vi "BonOMM-SAOMM.vi"() -> ()   [LabVIEW 2019] (continued)
          n252 = property on="Saturé" class="Bool (strict)"("Visible"=w229, "Blinking"=w229) -> ()  [unwired: 2 in, 2 out]
          n253 = call-poly <vilib>:"Read Key.vi"("section"=w271, "error in (no error)"=w284, "key"="DefaultROIOffset", "refnum"=w285) -> ("error out"=w276:errorcluster, "value"=w277:u32, "refnum out"=w275:T23)  [unwired: 4 in, 1 out]
          n254 = To Unsigned Word Integer(number=w333) -> (unsigned 16bit integer=w334:u16)
          n255 = To Unsigned Word Integer(number=w332) -> (unsigned 16bit integer=w331:u16)
          n256 = local write "ROIHeight"(w334) -> ()
          n257 = local write "ROIWidth"(w331) -> ()
          n258 = property on="TableXYPos" class="GraphXY (strict)"(error in=w535, "Active Cursor"=u32 1) -> (error out=w533:errorcluster)  [unwired: 1 in, 1 out]
          n259 = call-poly <vilib>:"Read Key.vi"("section"=w271, "error in (no error)"=w276, "key"="DefaultBinning", "refnum"=w275) -> ("error out"=w265:errorcluster, "value"=w278:u32, "refnum out"=w266:T23)  [unwired: 4 in, 1 out]
          n260 = call-poly <vilib>:"Read Key.vi"("section"=w260, "error in (no error)"=w265, "key"="GuideRateRA", "refnum"=w266) -> ("error out"=w351:errorcluster, "value"=w342:dbl, "refnum out"=w352:T23)  [unwired: 4 in, 1 out]
          n261 = local write "RateRA"(w342) -> ()
          n262 = call-poly <vilib>:"Read Key.vi"("section"=w260, "error in (no error)"=w351, "key"="GuideRateDEC", "refnum"=w352) -> ("error out"=w258:errorcluster, "value"=w341:dbl, "refnum out"=w259:T23)  [unwired: 4 in, 1 out]
          n263 = local write "RateDEC"(w341) -> ()
          n264 = call-poly <vilib>:"Read Key.vi"("section"=w260, "error in (no error)"=w258, "key"="HexXRate", "refnum"=w259) -> ("error out"=w264:errorcluster, "value"=w255:dbl, "refnum out"=w263:T23)  [unwired: 4 in, 1 out]
          n265 = local write "HexXRate"(w255) -> ()
          n266 = call-poly <vilib>:"Read Key.vi"("section"=w260, "error in (no error)"=w264, "key"="HexYRate", "refnum"=w263) -> ("error out"=w256:errorcluster, "value"=w254:dbl, "refnum out"=w257:T23)  [unwired: 4 in, 1 out]
          n267 = local write "HexYRate"(w254) -> ()
          n268 = call-poly <vilib>:"Read Key.vi"("section"=w260, "error in (no error)"=w256, "key"="BacklashRA", "refnum"=w257) -> ("error out"=w350:errorcluster, "value"=w340:dbl, "refnum out"=w353:T23)  [unwired: 4 in, 1 out]
          n269 = local write "BacklashRA"(w340) -> ()
          n270 = call-poly <vilib>:"Read Key.vi"("section"=w260, "error in (no error)"=w350, "key"="BacklashDEC", "refnum"=w353) -> ("error out"=w357:errorcluster, "value"=w339:dbl, "refnum out"=w356:T23)  [unwired: 4 in, 1 out]
          n271 = local write "BacklashDEC"(w339) -> ()
          n272 = call-poly <vilib>:"Read Key.vi"("section"=w260, "error in (no error)"=w357, "key"="GuiderAgg", "refnum"=w356) -> ("error out"=w355:errorcluster, "value"=w343:dbl, "refnum out"=w354:T23)  [unwired: 4 in, 1 out]
          n273 = local write "Corr%"(w343) -> ()
          n274 = call-poly <vilib>:"Read Key.vi"("section"=w260, "error in (no error)"=w355, "key"="GuiderTreshold", "refnum"=w354) -> ("error out"=w346:errorcluster, "value"=w344:dbl, "refnum out"=w347:T23)  [unwired: 4 in, 1 out]
          n275 = local write "CorrTreshold"(w344) -> ()
          n276 = call-poly <vilib>:"Read Key.vi"("section"=w260, "error in (no error)"=w346, "key"="SNRTreshold", "refnum"=w347) -> ("error out"=w267:errorcluster, "value"=→"SNRtreshold":dbl, "refnum out"=w268:T23)  [unwired: 4 in, 1 out]
          n277 = call-poly <vilib>:"Read Key.vi"("section"=w269, "error in (no error)"=w267, "key"="UAxisOffset", "refnum"=w268) -> ("error out"=w292:errorcluster, "value"=w287:dbl, "refnum out"=w293:T23)  [unwired: 4 in, 1 out]
          n278 = local write "DefaultUAxisOffset"(w287) -> ()
          n279 = call-poly <vilib>:"Read Key.vi"("section"=w269, "error in (no error)"=w292, "key"="VAxisOffset", "refnum"=w293) -> ("error out"=w290:errorcluster, "value"=w286:dbl, "refnum out"=w291:T23)  [unwired: 4 in, 1 out]
          n280 = local write "DefaultVAxisOffset"(w286) -> ()
          n281 = call-poly <vilib>:"Read Key.vi"("section"=w269, "error in (no error)"=w290, "key"="Sampling", "refnum"=w291) -> ("error out"=w327:errorcluster, "value"=→"Sampling rate":i32, "refnum out"=w328:T23)  [unwired: 4 in, 1 out]
          n282 = call-poly <vilib>:"Read Key.vi"("section"=w269, "error in (no error)"=w327, "key"="DataLenght", "refnum"=w328) -> ("error out"=w249:errorcluster, "value"=w345:i32, "refnum out"=w248:T23)  [unwired: 4 in, 1 out]
          n283 = local write "ConsideredLenght"(w345) -> ()
          n284 = local write "Flat"(w484) -> ()
          n285 = call-poly <vilib>:"Read Key.vi"("section"=w221, "error in (no error)"=w249, "key"="PRAMMS-SG", "refnum"=w248) -> ("error out"=w227:errorcluster, "value"=w246:u32, "refnum out"=w228:T23)  [unwired: 4 in, 1 out]
          n286 = property on="TableXYPos" class="GraphXY (strict)"(error in=w533, "Cursor.Cursor X"=w529, "Cursor.Cursor Y"=w529) -> ()  [unwired: 1 in, 2 out]
          n287 = local write "Néon"(w484) -> ()
          n288 = local write "Signature"(w246) -> ()
          n289 = To Unsigned Word Integer(number=w278) -> (unsigned 16bit integer=w279:u16)
          n290 = To Unsigned Word Integer(number=w277) -> (unsigned 16bit integer=w281:u16)
          n291 = To Unsigned Word Integer(number=w277) -> (unsigned 16bit integer=w280:u16)
          n292 = local write "Arc"(w484) -> ()
          n293 = local write "Binning"(w279) -> ()
          n294 = local write "ROIYOffset"(w281) -> ()
          n295 = local write "ROIXOffset"(w280) -> ()
          n296 = local write "NeonOn"(w484) -> ()
          n297 = local write "ArcOn"(w484) -> ()
          n298 = global read "Globals.vi" "BonOMM VI Refnum"() -> (w294:refnum<vi>)
          n299 = call-poly <vilib>:"Read Key.vi"("section"=w221, "error in (no error)"=w227, "key"="tempspd", "refnum"=w228) -> ("error out"=w224:errorcluster, "value"=w218:u32, "refnum out"=w225:T23)  [unwired: 4 in, 1 out]
          n300 = local write "FlatOn"(w484) -> ()
          n301 = Initialize Array(0.0, 0) -> (w252:dbl[])
          n302 = Initialize Array(sgl 0.0, w527, w527) -> (w526:sgl[][])
          n303 = Bundle(w424, w424, w424) -> (w423:cluster{string, string, string})  [unwired: 1 in]
          n304 = local write "ImgData"(w526) -> ()
          n305 = local write "MC_connect"(FALSE) -> ()
          n306 = call-poly <vilib>:"Read Key.vi"("section"=w221, "error in (no error)"=w224, "key"="tempvrn", "refnum"=w225) -> ("error out"=w222:errorcluster, "value"=w219:string, "refnum out"=w223:T23)  [unwired: 4 in, 1 out]
          n307 = call-poly <vilib>:"Read Key.vi"("section"=w313, "error in (no error)"=w222, "key"="xgain", "refnum"=w223) -> ("error out"=w320:errorcluster, "value"=→"Gain X":dbl, "refnum out"=w319:T23)  [unwired: 4 in, 1 out]
          n308 = call-poly <vilib>:"Read Key.vi"("section"=w313, "error in (no error)"=w320, "key"="ygain", "refnum"=w319) -> ("error out"=w315:errorcluster, "value"=→"Gain Y":dbl, "refnum out"=w316:T23)  [unwired: 4 in, 1 out]
          n309 = call-poly <vilib>:"Read Key.vi"("section"=w313, "error in (no error)"=w315, "key"="zgain", "refnum"=w316) -> ("error out"=w325:errorcluster, "value"=→"Gain Z":dbl, "refnum out"=w324:T23)  [unwired: 4 in, 1 out]
          n310 = call-poly <vilib>:"Read Key.vi"("section"=w313, "error in (no error)"=w325, "key"="ugain", "refnum"=w324) -> ("error out"=w323:errorcluster, "value"=→"Gain U":dbl, "refnum out"=w322:T23)  [unwired: 4 in, 1 out]
          n311 = call-poly <vilib>:"Read Key.vi"("section"=w313, "error in (no error)"=w323, "key"="vgain", "refnum"=w322) -> ("error out"=w273:errorcluster, "value"=→"Gain V":dbl, "refnum out"=w274:T23)  [unwired: 4 in, 1 out]
          n312 = call-poly <vilib>:"Read Key.vi"("section"="options", "error in (no error)"=w273, "default value"=FALSE, "key"="autoconnect", "refnum"=w274) -> ("error out"=w389:errorcluster, "value"=w385:bool, "refnum out"=w390:T23)  [unwired: 3 in, 1 out]
          n313 = local write "AutoConnect?"(w385) -> ()
          n314 = call-poly <vilib>:"Read Key.vi"("section"=w393, "error in (no error)"=w389, "key"="secperpulse", "refnum"=w390) -> ("error out"=w403:errorcluster, "value"=w242:dbl, "refnum out"=w405:T23)  [unwired: 4 in, 1 out]
          "arcsec/pulse" <- w242
          n315 = call-poly <vilib>:"Read Key.vi"("section"=w393, "error in (no error)"=w403, "key"="naxis1", "refnum"=w405) -> ("error out"=w402:errorcluster, "value"=w243:dbl, "refnum out"=w404:T23)  [unwired: 4 in, 1 out]
          n316 = local write "NaxisMax"(w243) -> ()
          n317 = Multiply(x=w243, y=w242) -> (x*y=w241:dbl)
          n318 = call-poly <vilib>:"Read Key.vi"("section"=w393, "error in (no error)"=w402, "key"="represent", "refnum"=w404) -> ("error out"=w434:errorcluster, "value"=w431:dbl, "refnum out"=w435:T23)  [unwired: 4 in, 1 out]
          "Représentation" <- w431
          n319 = expression code="x/60"(w241) -> (→"RangeTable":dbl)
          n320 = call-poly <vilib>:"Read Key.vi"("section"=w393, "error in (no error)"=w434, "key"="cenx", "refnum"=w435) -> ("error out"=w516:errorcluster, "value"=w515:i32, "refnum out"=w517:T23)  [unwired: 4 in, 1 out]
          n321 = local write "CentreTel X"(w515) -> ()
          n322 = call-poly <vilib>:"Read Key.vi"("section"=w393, "error in (no error)"=w516, "key"="ceny", "refnum"=w517) -> ("error out"=w508:errorcluster, "value"=w514:i32, "refnum out"=w509:T23)  [unwired: 4 in, 1 out]
          n323 = local write "CentreTel Y"(w514) -> ()
          n324 = call-poly <vilib>:"Read Key.vi"("section"=w393, "error in (no error)"=w508, "key"="refx", "refnum"=w509) -> ("error out"=w513:errorcluster, "value"=w507:i32, "refnum out"=w512:T23)  [unwired: 4 in, 1 out]
          n325 = local write "Reference X"(w507) -> ()
          n326 = call-poly <vilib>:"Read Key.vi"("section"=w393, "error in (no error)"=w513, "key"="refy", "refnum"=w512) -> ("error out"=w444:errorcluster, "value"=w506:i32, "refnum out"=w445:T23)  [unwired: 4 in, 1 out]
          n327 = local write "Reference Y"(w506) -> ()
          n328 = Less Or Equal?(x=w431, y=70.0) -> (x <= y?=w429:bool)
          n329 = call-poly <vilib>:"Read Key.vi"("section"=w393, "error in (no error)"=w444, "key"="rangex", "refnum"=w445) -> ("error out"=w446:errorcluster, "value"=w449:i32, "refnum out"=w447:T23)  [unwired: 4 in, 1 out]
          n330 = local write "Rangement X"(w449) -> ()
          n331 = Select(t=T17."Enabled" ("Disabled"), s=w429, f=T17."Disabled" ("Disabled")) -> (s? t:f=w426:T17)
          n332 = call-poly <vilib>:"Read Key.vi"("section"=w393, "error in (no error)"=w446, "key"="rangey", "refnum"=w447) -> ("error out"=w440:errorcluster, "value"=w450:i32, "refnum out"=w441:T23)  [unwired: 4 in, 1 out]
          n333 = local write "Rangement Y"(w450) -> ()
          n334 = property on="GetDSS" class="Bool (strict)"("DisabledEnum"=w426) -> ()  [unwired: 2 in, 2 out]
          n335 = call-poly <vilib>:"Read Key.vi"("section"=w393, "error in (no error)"=w440, "key"="rangez", "refnum"=w441) -> ("error out"=w438:errorcluster, "value"=w437:i32, "refnum out"=w439:T23)  [unwired: 4 in, 1 out]
          n336 = local write "Rangement Z"(w437) -> ()
          n337 = call-poly <vilib>:"Read Key.vi"("section"=w393, "error in (no error)"=w438, "key"="vrapid", "refnum"=w439) -> ("error out"=w476:errorcluster, "value"=→"vitesse rapide":dbl, "refnum out"=w475:T23)  [unwired: 4 in, 1 out]
          n338 = call-poly <vilib>:"Read Key.vi"("section"=w393, "error in (no error)"=w476, "key"="vlente", "refnum"=w475) -> ("error out"=w482:errorcluster, "value"=→"vitesse lente":dbl, "refnum out"=w481:T23)  [unwired: 4 in, 1 out]
          n339 = call-poly <vilib>:"Read Key.vi"("section"=w393, "error in (no error)"=w482, "key"="accel", "refnum"=w481) -> ("error out"=w477:errorcluster, "value"=→"accelleration":dbl, "refnum out"=w478:T23)  [unwired: 4 in, 1 out]
          n340 = call-poly <vilib>:"Read Key.vi"("section"=w393, "error in (no error)"=w477, "key"="vfocus", "refnum"=w478) -> ("error out"=w396:errorcluster, "value"=→"vitesse focus":dbl, "refnum out"=w397:T23)  [unwired: 4 in, 1 out]
          n341 = call-poly <vilib>:"Read Key.vi"("section"=w393, "error in (no error)"=w396, "key"="vjog", "refnum"=w397) -> ("error out"=w394:errorcluster, "value"=→"vitesse jog":dbl, "refnum out"=w395:T23)  [unwired: 4 in, 1 out]
          n342 = call <vilib>:"Close Config Data.vi"("error in (no error)"=w394, "refnum"=w395) -> ("file path"=w454:path)  [unwired: 8 in, 1 out]
          n343 = call "Readwindowpropfile.vi"("configuration file path"=w454) -> ("PanelOrigin"=w296:cluster{"panelx":i16, "panely":i16}, "MinimumSize"=w297:cluster{"Horizontal":i16, "Vertical":i16}, "PanelBounds"=w298:T24, "resizable"=w299:bool, "AllFound"=w295:bool)  [unwired: 6 in]
          n344 = Bundle(w252, w252) -> (w460:cluster{dbl[], dbl[]})  [unwired: 1 in]
          n345 = Initialize Array(w423, 0) -> (→"CmdDone":cluster{string, string, string}[])
          n346 = flat-sequence {
            tunnel: w294 -> [w569]
            tunnel: w299 -> [w570]
            tunnel: w298 -> [w571]
            tunnel: w297 -> [w565]
            tunnel: [w572] -> w306
            tunnel: w296 -> [w572]
            tunnel: [w568] -> w305
            tunnel: [w571] -> w304
            tunnel: [w570] -> w303
            tunnel: [w566] -> w302
            tunnel: [w565] -> w301
            tunnel: w306 -> [w578]
            tunnel: [w578] -> w300
            tunnel: w305 -> [w577]
            tunnel: w304 -> [w576]
            tunnel: w303 -> [_]
            tunnel: w302 -> [w575]
            tunnel: w301 -> [w574]
            tunnel: w300 -> [w584]
            frame #0 {
              n347 = property class="VI"(reference=w569, "Front Panel.Resizeable"=TRUE ("Front Panel Window:Resizable")) -> (reference out=w568:refnum<vi>, error out=w566:errorcluster)  [unwired: 1 in]
            }
            frame #1 {
              n348 = disable-structure shown="Disabled" {
                disable-tunnel: w577 -> [w583 _]
                disable-tunnel: w576 -> [w582 _]
                disable-tunnel: w575 -> [w581 _]
                disable-tunnel: w574 -> [w580 _]
                disable-tunnel: TRUE ("Front Panel Window:Resizable") -> [w579 _]
                frame Disabled {
                  n349 = property class="VI"(reference=w583, error in=w581, "Front Panel.Resizeable"=w579, "Front Panel.PanelBounds"=w582, "Minimum Panel Size"=w580) -> ()  [unwired: 2 out]
                }
                frame Enabled {
                }
              }
            }
            frame #2 {
              n350 = property on="Pane" class="Pann"("Origin"=w584) -> ()  [unwired: 2 in, 2 out]
              n351 = property on="MainTab" class="Onglet (strict)"("Position"=cluster{i32, i32} {0, 0}) -> ()  [unwired: 2 in, 2 out]
            }
            frame #3 {
              "Lecture Configuration" <- TRUE ("Lecture Configuration")
            }
          }
          n352 = case shown="Vrai" w295 {
            frame False {
              # "Ne devrais pas arriver ..."
              n353 = One Button Dialog(message="Impossible de trouver le fichier properties.ini\nUtilisation des valeurs par défauts ...") -> ()  [unwired: 1 in, 1 out]
            }
            frame True {
            }
          }
          n354 = local write "LVDT-RA-Data"(w252) -> ()
          n355 = call "Draw_crosshair.vi"("Image IN"=w526, "White Value"=sgl 255.0) -> ("Image OUT"=w525:sgl[][])  [unwired: 13 in]
          n356 = Initialize Array(w460, 0) -> (w253:cluster{dbl[], dbl[]}[])
          n357 = Initialize Array("", 0) -> (w469:string[])
          n358 = Initialize Array(refnum<k5> refnum ("External TCP ID 2"), 0) -> (w467:refnum<k5>[])
          n359 = local write "subimg"(w525) -> ()
          n360 = local write "Img DEC"(w436) -> ()
          n361 = local write "RA-USNO"(w436) -> ()
          n362 = local write "DEC-USNO"(w436) -> ()
          n363 = local write "Img RA"(w436) -> ()
          n364 = local write "Graph-Flux"(w253) -> ()
          n365 = local write "Graph-Centroids"(w253) -> ()
          n366 = local write "Graph-SNR"(w253) -> ()
          n367 = local write "ImageUsage"(w384) -> ()
          n368 = disable-structure shown="Activé" {
            disable-tunnel: w219 -> [w563 _]
            disable-tunnel: w218 -> [w562 _]
            frame Disabled {
              n369 = Type Cast(type=refnum<visa-resource-name> "-1" ("Table VRN"), x=w563) -> (*(type *) &x=w557:refnum<visa-resource-name>)
              n370 = local write "HexTemp Baud rate"(w562) -> ()
              n371 = local write "HexTemp VRN"(w557) -> ()
              n372 = call-poly "VISA Configure Serial Port"("VISA resource name"=w557, "timeout (10sec)"=u32 1000, "Enable Termination\nChar (T)"=FALSE ("Enable Termination\nChar (T)"), "baud rate (9600)"=w562) -> ("error out"=w558:errorcluster)  [unwired: 10 in, 1 out]
              n373 = local write "HexapodeTempError"(w558) -> ()
            }
            frame Enabled {
            }
          }
          n374 = local write "Clients ID"(w467) -> ()
          n375 = local write "Clients"(w469) -> ()
          n376 = local write "Hex-XGraph"(w253) -> ()
          n377 = local write "Guiderreur"(w253) -> ()
          n378 = local write "Hex-YGraph"(w253) -> ()
          n379 = local write "Cumulatif"(w253) -> ()
          n380 = local write "CumulativeError"(w253) -> ()
          n381 = local write "CentroidsData"(w253) -> ()
          n382 = local write "HexXData"(w253) -> ()
          n383 = local write "HexYData"(w253) -> ()
          n384 = local write "SNRData"(w253) -> ()
          n385 = local write "FluxData"(w253) -> ()
          "RAtmp" <- w436
          "Dectmp" <- w436
          "Menu Error" <- w472
          "VI Reference Error" <- w472
          "Starry Night Error" <- w472
          "Excom Error" <- w472
          "Guider Error" <- w472
          "ActiveX Error" <- w472
          "Critical Error" <- w472
          "Config Error" <- w472
          "Serial Error" <- w472
          "TCP/IP Error" <- w472
          "wget error" <- w472
          "TCS Error" <- w472
          "File I/O Error" <- w472
          "FIFO actif" <- w244
          "TCS actif" <- w244
          "TCS C actif" <- w244
          "Table actif" <- w244
          "Integrating" <- w244
          "MovingXY" <- w244
          "MovingZ" <- w244
          "CorrectZ" <- w244
          "CorrectXY" <- w244
          "Focusing" <- w244
          "CurvCorrect" <- w244
          "SubIMG4DSS?" <- w244
          "AS_I_Pillier" <- FALSE ("AS_Pillier")
          "GE_TCS" <- FALSE ("GE_TCS")
        }
      }
      n386 = property on="Déc étoile guide" class="NumNb (strict)"("Visible"=w201) -> ()  [unwired: 2 in, 2 out]
      n387 = property on="A.D. étoile guide" class="NumNb (strict)"("Visible"=w201) -> ()  [unwired: 2 in, 2 out]
      n388 = property on="Graph-Centroids" class="GraphXY (strict)"("Visible"=w201) -> ()  [unwired: 2 in, 2 out]
      n389 = property on="Flux Max" class="NumNb (strict)"("Visible"=w201) -> ()  [unwired: 2 in, 2 out]
      n390 = property on="Guiderreur" class="GraphXY (strict)"("Visible"=w201) -> ()  [unwired: 2 in, 2 out]
      n391 = property on="Flux inst." class="NumNb (strict)"("Visible"=w201) -> ()  [unwired: 2 in, 2 out]
      n392 = property on="StopCam" class="Bool (strict)"("Visible"=w201) -> ()  [unwired: 2 in, 2 out]
      n393 = property on="GoCam" class="Bool (strict)"("Visible"=w201) -> ()  [unwired: 2 in, 2 out]
      n394 = property on="Approaching limit" class="Bool (strict)"("Visible"=w203, "Blinking"=w203) -> ()  [unwired: 2 in, 2 out]
      n395 = property on="Target OutofRange" class="Bool (strict)"("Visible"=w203, "Blinking"=w203) -> ()  [unwired: 2 in, 2 out]
      n396 = property on="Lampe Allumée ?" class="Bool (strict)"("Visible"=w203, "Blinking"=w203) -> ()  [unwired: 2 in, 2 out]
      n397 = property on="ModeInv" class="Bool (strict)"("Visible"=w203, "Blinking"=w203) -> ()  [unwired: 2 in, 2 out]
      n398 = property on="StarFaded?" class="Bool (strict)"("Visible"=w203, "Blinking"=w203) -> ()  [unwired: 2 in, 2 out]
      n399 = property on="Alarme PRAMS" class="Bool (strict)"("Visible"=w203, "Blinking"=w203) -> ()  [unwired: 2 in, 2 out]
      n400 = property on="Picture" class="Image"("Visible"=w202) -> ()  [unwired: 2 in, 2 out]
      n401 = property on="filtre_nom" class="Ch"("Visible"=w202) -> ()  [unwired: 2 in, 2 out]
      n402 = property on="q-raf" class="Bool (strict)"("Visible"=w202) -> ()  [unwired: 2 in, 2 out]
      n403 = property on="cancel-raf" class="Bool (strict)"("Visible"=w202) -> ()  [unwired: 2 in, 2 out]
      n404 = property on="change_filtre_liste" class="Bool (strict)"("Visible"=w202) -> ()  [unwired: 2 in, 2 out]
      n405 = property on="ChoixFiltre" class="Clust (strict)"("Visible"=w202) -> ()  [unwired: 2 in, 2 out]
      n406 = property on="F#" class="NumNb (strict)"("Visible"=w202) -> ()  [unwired: 2 in, 2 out]
      n407 = property on="ST-" class="Bool (strict)"("Visible"=w202) -> ()  [unwired: 2 in, 2 out]
      n408 = property on="ST+" class="Bool (strict)"("Visible"=w202) -> ()  [unwired: 2 in, 2 out]
      n409 = property on="SET ZERO" class="Bool"("Visible"=w202) -> ()  [unwired: 2 in, 2 out]
      n410 = property on="ST_RAZ" class="Bool"("Visible"=w202) -> ()  [unwired: 2 in, 2 out]
      n411 = property on="reconnect" class="Bool (strict)"("Visible"=w202) -> ()  [unwired: 2 in, 2 out]
      n412 = property on="ST_SPD" class="Gliss (strict)"("Visible"=w202) -> ()  [unwired: 2 in, 2 out]
      "GE_Hex_X" <- w200
      "GE_Hex_Y" <- w200
      "GE_Hex_Z" <- w200
      "GE_Hex_U" <- w200
      "GE_Hex_V" <- w200
    }
    frame #4 {
      # "Étape 4 de l'initialisation"
      # "Initialisation des éléments du menu"
      n413 = case shown="Vrai" w587 {
        frame False {
        }
        frame True {
          w671 = refnum<visa-resource-name> "-1" ("Table VRN")
          # "Menu \"FA (Fonctions avancées)\""
          # "Désactive les filtres"
          # "Menu \"Roue à filtre\""
          # "Menu \"Tables de guidage\""
          # "Menu \"Caméra de référence\""
          # "Menu \"Secondaire Actif\""
          # "Menu \"Télescope\""
          # "Menu des scripts"
          # "Menu des Instruments"
          # "Menu des communications"
          # "Ajoute les items de menu custom"
          # "Enlève les items de menu non-utilisés"
          n414 = Current VI's Menubar ("Barre de menu")() -> (w715:refnum<k9>)
          n415 = Delete Menu Items(7:string[] ["APP_EDIT", "APP_VIEW", "APP_PROJECT", "APP_TOOLS"], 9:w715) -> (0:w673:errorcluster, 3:w674:refnum<k9>)  [unwired: 2 in]
          n416 = call "MenuFixer.vi"("Menu Name"=string[] ["Communications", "Instruments", "Scripts et Automatismes", "Télescope", "Secondaire Actif", "Caméra de référence", "Tables de guidage", "Roue à filtres", "FA"] ("Array Constant"), "Prefix"="main_") -> ("Item Tags"=w614:string[], "Item Names"=w613:string[])  [unwired: 8 in]
          n417 = call "MenuFixer.vi"("Menu Name"=string[] ["Charger la librairie CPAPIR", "Charger la librairie Pesto", "Charger une librairie d'objets", "APP_SEPARATOR", "Déterminer l'astrométrie du champ", "Calibration du foyer automatique", "APP_SEPARATOR", "Construction d'une LUT"] ("menuelem_cmd"), "Prefix"="scp_") -> ("Item Tags"=w626:string[], "Item Names"=w625:string[])  [unwired: 8 in]
          n418 = Insert Menu Items(4:"APP_OPERATE" ("after item"), 6:w673, 7:w614, 8:w613, 9:w674) -> (0:w664:errorcluster, 3:w665:refnum<k9>)  [unwired: 1 in, 1 out]
          n419 = call "MenuFixer.vi"("Menu Name"=string[] ["Telescope Control System", "Caméra de référence", "Tables de guidage", "Secondaire Actif", "Module de calibration", "MC-BonOMM", "Commandes externes", "Station Météo", "APP_SEPARATOR", "Reconnexion automatique ?"] ("menu_comm"), "Prefix"="com_") -> ("Item Tags"=w612:string[], "Item Names"=w618:string[])  [unwired: 8 in]
          n420 = Insert Menu Items(5:"main_Communications" ("menu tag"), 6:w664, 7:w612, 8:w618, 9:w665) -> (0:w707:errorcluster, 3:w708:refnum<k9>)  [unwired: 1 in, 1 out]
          n421 = call "MenuFixer.vi"("Menu Name"=string[] ["Synchroniser la coupole", "Synchroniser les horloges", "Modifier la vitesse du télescope", "Modifier la vitesse de guidage", "Modifier l'époque d'affichage", "Test signal vers TCS ", "APP_SEPARATOR", "Reconnexion"] ("menuelem_cmd"), "Prefix"="tel_") -> ("Item Tags"=w631:string[], "Item Names"=w630:string[])  [unwired: 8 in]
          n422 = Index Array(array=w612) -> (element #1=w698:string, element #2=w697:string, element #3=w696:string, element #4=w666:string, element #5=w679:string, element #6=w678:string, element #7=w677:string, element #8=w676:string, element #10=w675:string)  [unwired: 10 in, 1 out]
          n423 = local read "TCS VRN"() -> (w704:refnum<visa-resource-name>)
          n424 = Not Equal?(x=w704, y=w671) -> (x != y?=w689:bool)
          n425 = local write "TCS COMM"(w689) -> ()
          n426 = Set Menu Item Info(6:w689, 7:w698, 8:w707, 11:w708) -> (0:w710:errorcluster, 3:w709:refnum<k9>)  [unwired: 3 in]
          n427 = local read "PrAMS VRN"() -> (w703:refnum<visa-resource-name>)
          n428 = Not Equal?(x=w703, y=w671) -> (x != y?=w688:bool)
          n429 = local write "PrAMS COMM"(w688) -> ()
          n430 = Set Menu Item Info(6:w688, 7:w697, 8:w710, 11:w709) -> (0:w712:errorcluster, 3:w711:refnum<k9>)  [unwired: 3 in]
          n431 = local read "Table VRN"() -> (w702:refnum<visa-resource-name>)
          n432 = call "MenuFixer.vi"("Menu Name"=string[] ["Paramètres d'asservissement", "Commander l'hexapode", "Panneau de offset", "Déplacement manuel", "APP_SEPARATOR", "Remise à zéro", "APP_SEPARATOR", "Reconnexion"] ("menuelem_cmd"), "Prefix"="hex_") -> ("Item Tags"=w635:string[], "Item Names"=w634:string[])  [unwired: 8 in]
          n433 = Not Equal?(x=w702, y=w671) -> (x != y?=w687:bool)
          n434 = local write "TableCOM"(w687) -> ()
          n435 = Set Menu Item Info(6:w687, 7:w696, 8:w712, 11:w711) -> (0:w667:errorcluster, 3:w670:refnum<k9>)  [unwired: 3 in]
          n436 = local read "Hexapod VRN"() -> (w672:refnum<visa-resource-name>)
          n437 = Not Equal?(x=w672, y=w671) -> (x != y?=w645:bool)
          n438 = local write "Hexapod COMM"(w645) -> ()
          n439 = Set Menu Item Info(6:w645, 7:w666, 8:w667, 11:w670) -> (0:w668:errorcluster, 3:w669:refnum<k9>)  [unwired: 3 in]
          n440 = local read "Calib VRN"() -> (w701:refnum<visa-resource-name>)
          n441 = Not Equal?(x=w701, y=w671) -> (x != y?=w684:bool)
          n442 = local write "Calib COMM"(w684) -> ()
          n443 = Set Menu Item Info(6:w684, 7:w679, 8:w668, 11:w669) -> (0:w714:errorcluster, 3:w713:refnum<k9>)  [unwired: 3 in]
          n444 = local read "MC-BonOMM VRN"() -> (w700:refnum<visa-resource-name>)
          n445 = call "MenuFixer.vi"("Menu Name"=string[] ["Enregistrer la prochaine image", "Modifier les paramètres", "Modifier la région d'intérêt", "APP_SEPARATOR", "Binning 1x1", "Binning 2x2", "Binning 4x4", "Binning 5x5", "APP_SEPARATOR", "Reconnexion"] ("menuelem_cmd"), "Prefix"="cam_") -> ("Item Tags"=w640:string[], "Item Names"=w639:string[])  [unwired: 8 in]
          n446 = Not Equal?(x=w700, y=w671) -> (x != y?=w685:bool)
          n447 = local write "MCB COMM"(w685) -> ()
          n448 = Set Menu Item Info(6:w685, 7:w678, 8:w714, 11:w713) -> (0:w705:errorcluster, 3:w706:refnum<k9>)  [unwired: 3 in]
          n449 = local read "Excmd VRN"() -> (w699:refnum<visa-resource-name>)
          n450 = Not Equal?(x=w699, y=w671) -> (x != y?=w686:bool)
          n451 = Set Menu Item Info(6:w686, 7:w677, 8:w705, 11:w706) -> (0:w694:errorcluster, 3:w695:refnum<k9>)  [unwired: 3 in]
          n452 = local write "ExCmd COMM"(w686) -> ()
          n453 = local read "Cx"() -> (w693:bool)
          n454 = local read "AutoConnect?"() -> (w682:bool)
          n455 = Set Menu Item Info(6:w693, 7:w676, 8:w694, 11:w695) -> (0:w680:errorcluster, 3:w681:refnum<k9>)  [unwired: 3 in]
          n456 = call "MenuFixer.vi"("Menu Name"=string[] ["Mode Guidage et Dither", "", "", "", "", "", ""] ("menuelem_cmd"), "Prefix"="fa_") -> ("Item Tags"=w594:string[], "Item Names"=w598:string[])  [unwired: 8 in]
          n457 = local read "Mode Guidage et Dither"() -> (w588:bool)
          n458 = call "MenuFixer.vi"("Menu Name"=string[] ["Modifier les vitesses des tables", "Positions prédéfinies", "Commandes XYZ", "APP_SEPARATOR", "Modifier les paramètres", "APP_SEPARATOR", "Reconnexion"] ("menuelem_cmd"), "Prefix"="tab_") -> ("Item Tags"=w644:string[], "Item Names"=w643:string[])  [unwired: 8 in]
          n459 = Set Menu Item Info(6:w682, 7:w675, 8:w680, 11:w681) -> (0:w683:errorcluster, 3:w621:refnum<k9>)  [unwired: 3 in]
          n460 = Index Array(array=w594) -> (element #1=w589:string)  [unwired: 10 in, 9 out]
          n461 = local read "instruments.ini"() -> (w690:path)
          n462 = local read "Tableau des filtres"() -> (w601:string[])
          n463 = call "RaFMenuFixer.vi"("Tableau des filtres"=w601, "Prefix"="raf_") -> ("Item Tags"=w602:string[], "Item Names"=w603:string[])  [unwired: 8 in]
          n464 = call <vilib>:"Open Config Data.vi"("create file if necessary (T)"=FALSE, "configuration file path"=w690) -> ("error out"=w721:errorcluster, "refnum"=w722:T23)  [unwired: 7 in, 1 out]
          n465 = Array Size(array=w601) -> (size(s)=w608:i32)
          n466 = call <vilib>:"Get Section Names.vi"("error in (no error)"=w721, "refnum"=w722) -> ("error out"=w716:errorcluster, "section names"=w691:string[], "refnum out"=w717:T23)  [unwired: 7 in]
          "section names" <- w691
          n467 = Array Subset(array=w602, index=2, length=w608) -> (w605:string[])
          n468 = Array Subset(array=w603, index=2, length=w608) -> (w604:string[])
          n469 = call <vilib>:"Close Config Data.vi"("error in (no error)"=w716, "refnum"=w717) -> ()  [unwired: 8 in, 2 out]
          n470 = Build Array (concatenate)(w691, "APP_SEPARATOR", "Modifier les paramètres") -> (w623:string[])
          n471 = call "MenuFixer.vi"("Menu Name"=w623, "Prefix"="ins_") -> ("Item Tags"=w622:string[], "Item Names"=w620:string[])  [unwired: 8 in]
          n472 = Insert Menu Items(5:"main_Instruments" ("menu tag"), 6:w683, 7:w622, 8:w620, 9:w621) -> (0:w658:errorcluster, 3:w659:refnum<k9>)  [unwired: 1 in, 1 out]
          n473 = Insert Menu Items(5:"main_Scripts et Automatismes" ("menu tag"), 6:w658, 7:w626, 8:w625, 9:w659) -> (0:w660:errorcluster, 3:w661:refnum<k9>)  [unwired: 1 in, 1 out]
          n474 = Insert Menu Items(5:"main_Télescope" ("menu tag"), 6:w660, 7:w631, 8:w630, 9:w661) -> (0:w655:errorcluster, 3:w656:refnum<k9>)  [unwired: 1 in, 1 out]
          n475 = Insert Menu Items(5:"main_Secondaire Actif" ("menu tag"), 6:w655, 7:w635, 8:w634, 9:w656) -> (0:w652:errorcluster, 3:w653:refnum<k9>)  [unwired: 1 in, 1 out]
          n476 = Insert Menu Items(5:"main_Caméra de référence" ("menu tag"), 6:w652, 7:w640, 8:w639, 9:w653) -> (0:w649:errorcluster, 3:w650:refnum<k9>)  [unwired: 1 in, 1 out]
          n477 = Insert Menu Items(5:"main_Tables de guidage " ("menu tag"), 6:w649, 7:w644, 8:w643, 9:w650) -> (0:w646:errorcluster, 3:w647:refnum<k9>)  [unwired: 1 in, 1 out]
          n478 = Insert Menu Items(5:"main_Roue à filtres" ("menu tag"), 6:w646, 7:w602, 8:w603, 9:w647) -> (0:w610:errorcluster, 3:w611:refnum<k9>)  [unwired: 1 in, 1 out]
          n479 = for {
            tunnel: [w730] -> w595
            tunnel: w611 -> [w732]
            tunnel: w610 -> [w731]
            tunnel: [w729] -> w596
            tunnel: w605 -> [w727] mode=indexing
            tunnel: w604 -> [w726] mode=indexing
            w728 = FALSE ("enabled")
            n480 = Set Menu Item Info(6:w728, 7:w727, 8:w731, 9:w728, 10:w726, 11:w732) -> (0:w729:errorcluster, 3:w730:refnum<k9>)  [unwired: 1 in]
          }
          n481 = Insert Menu Items(5:"main_FA" ("menu tag"), 6:w596, 7:w594, 8:w598, 9:w595) -> (0:w593:errorcluster, 3:w592:refnum<k9>)  [unwired: 1 in, 1 out]
          n482 = Set Menu Item Info(6:w588, 7:w589, 8:w593, 11:w592) -> (0:w591:errorcluster, 3:w590:refnum<k9>)  [unwired: 3 in]
          n483 = flat-sequence {
            tunnel: w590 -> [w733]
            tunnel: w591 -> [w734]
            tunnel: [w733] -> _
            frame #0 {
              n484 = local write "Menu Error"(w734) -> ()
              "menu ref" <- w733
            }
            frame #1 {
              "Gestion des menus" <- TRUE ("Gestion des menus")
            }
          }
        }
      }
    }
    frame #5 {
      # "Étape 5 de l'initialisation"
      # "Initialisation de SAOMM"
      n485 = case shown="Vrai" w736 {
        frame False {
        }
        frame True {
          n486 = flat-sequence {
            tunnel: [TRUE] -> w737
            frame #0 {
              w740 = 0 ("Signature")
              w742 = 0 ("Nb_ACK")
              w738 = FALSE ("PRAMMS actif")
              # "Mettre dans le fichier de configuration ..."
              # "Signature Sale ..."
              n487 = local read "path_config"() -> (w750:path)
              n488 = Build Path(base path=w750, name or relative path=path "command.ini" ("command.ini")) -> (appended path=w748:path)
              n489 = call "SAOMM-BuildTypeArray.vi"("command.ini"=w748) -> ("CommandArray"=→"MessageType":cluster{string[], u32[]})  [unwired: 14 in]
              n490 = local write "Signature"(u32 1886544237 ("Signature")) -> ()
              n491 = local write "PrAMS-ACK"(w740) -> ()
              n492 = local write "Hexapod-ACK"(w740) -> ()
              n493 = local write "LastProcSavedID"(u64 0 ("LastProcSavedID")) -> ()
              n494 = local read "properties.ini"() -> (w746:path)
              n495 = local write "Nb_ACK (PrAMS)"(w742) -> ()
              n496 = local write "Nb_ACK (hex)"(w742) -> ()
              n497 = local write "Nb_Error (PrAMS)"(w742) -> ()
              n498 = local write "Nb_Error (hex)"(w742) -> ()
              n499 = local write "ImgArray"(u32[][] [] ("ImgArray")) -> ()
              n500 = call "SAOMM-ROIEnums.vi"("Path"=w746) -> ("StringEnums"=w745:string[], "ROISizes"=→"ROISizes":i32[])  [unwired: 13 in]
              n501 = local write "CorrDelay"(u32 5000 ("CorrDelay")) -> ()
              n502 = local write "QueryingHexapod"(w738) -> ()
              n503 = local write "PrAMS-Error"(w738) -> ()
              n504 = local write "Servo"(w738) -> ()
              n505 = local write "HexaCons actif"(w738) -> ()
              n506 = local write "Hexapod-Error"(w738) -> ()
              n507 = local write "LastProcID"(u64 0 ("Last Received ID")) -> ()
              n508 = property on="ROIsurface" class="MDér (strict)"("Strings []"=w745) -> ()  [unwired: 2 in, 2 out]
              "PrAMS Error" <- errorcluster {"status"=FALSE, "code"=0, "source"=""} ("PRAMMS Error")
              "PrAMS actif" <- w738
              "HxMoving" <- w738
              "Exceptions" <- T19 {"Command Error"=FALSE, "Slip/Stall"=FALSE, "Overtravel"=FALSE, "Done"=FALSE, "nError"=0.0, "nSlip"=0.0, "nOT"=0.0, "nDone"=0.0} ("Newmark-Exceptions")
              "Guidage en cour" <- w738
            }
            frame #1 {
              w757 = T17."Enabled" ("Disabled")
              w758 = T17."Disabled and Grayed Out" ("Disabled")
              w760 = u16 2 items=["Opération Fixe", "Asservissement Ouvert", "Asservissement Fermé", "Calibration"] ("Mode")
              w756 = u32 0 ("ListenerExec")
              w761 = u16 2 items=["1 x 1"=1, "2 x 2"=2, "4 x 4"=4, "5 x 5"=5] ("Binning")
              n509 = local write "GetOptimalTime"(w756) -> ()
              n510 = local write "GetOptimalTime"(w756) -> ()
              n511 = local write "Nb_FalconProc_demandé"(w756) -> ()
              n512 = local write "SetBinningTime"(w756) -> ()
              n513 = local write "Nb_FalconProc_reçu"(w756) -> ()
              n514 = local write "SetFPSTime"(w756) -> ()
              n515 = local write "SetROITime"(w756) -> ()
              n516 = local write "StopTime"(w756) -> ()
              n517 = local write "FalconQuery"(w756) -> ()
              n518 = local write "HexapodQuery"(w756) -> ()
              n519 = local write "ListenerExec"(w756) -> ()
              n520 = local write "SetExpTime"(w756) -> ()
              n521 = local write "StartTime"(w756) -> ()
              n522 = local write "Dump"("" ("Dump")) -> ()
              n523 = local write "Binning"(w761) -> ()
              n524 = local write "Mode"(w760) -> ()
              n525 = property on="GoCam" class="Bool (strict)"("DisabledEnum"=w757) -> ()  [unwired: 2 in, 2 out]
              n526 = property on="StopCam" class="Bool (strict)"("DisabledEnum"=w757) -> ()  [unwired: 2 in, 2 out]
              n527 = property on="XReference" class="NumNb (strict)"("DisabledEnum"=w757) -> ()  [unwired: 2 in, 2 out]
              n528 = property on="YReference" class="NumNb (strict)"("DisabledEnum"=w757) -> ()  [unwired: 2 in, 2 out]
              n529 = property on="StartServo" class="Bool (strict)"("DisabledEnum"=w758) -> ()  [unwired: 2 in, 2 out]
              n530 = property on="StopServo" class="Bool (strict)"("DisabledEnum"=w758) -> ()  [unwired: 2 in, 2 out]
              n531 = property on="Mode" class="MDér (strict)"("DisabledEnum"=T17."Enabled" ("Disabled")) -> ()  [unwired: 2 in, 2 out]
            }
            frame #2 {
              w762 = -1.0 ("LastImageTime")
              # "Initialisation des tableaux de données ..."
              n532 = local read "properties.ini"() -> (w771:path)
              n533 = Initialize Array(-inf ("LastImageTime"), 5 ("dimension size")) -> (w786:dbl[])
              n534 = local read "path_config"() -> (w764:path)
              n535 = local write "FalconProcTimeStamp"(w762) -> ()
              n536 = local write "LastImageTime"(w762) -> ()
              n537 = local write "LastSaveTimeStamp"(w762) -> ()
              n538 = call <vilib>:"Open Config Data.vi"("create file if necessary (T)"=FALSE, "configuration file path"=w771) -> ("error out"=w769:errorcluster, "refnum"=w768:T23)  [unwired: 7 in, 1 out]
              n539 = local read "Signature"() -> (w784:u32)
              n540 = local write "H_LUT"(w786) -> ()
              n541 = local write "H_Offset"(w786) -> ()
              n542 = local write "H_Servo"(w786) -> ()
              n543 = local write "H_Console"(w786) -> ()
              n544 = local write "H_Position"(w786) -> ()
              n545 = Build Path(base path=w764, name or relative path=path "command.ini" ("command.ini")) -> (appended path=w763:path)
              n546 = call-poly <vilib>:"Read Key.vi"("section"="communications" ("key"), "error in (no error)"=w769, "key"="PRAMMS-IP", "refnum"=w768) -> ("error out"=w775:errorcluster, "value"=w767:string, "refnum out"=w774:T23)  [unwired: 4 in, 1 out]
              n547 = call "Hexapod-connect.vi"("IP"=w767, "Port"=u16 10010, "Signature"=w784, "path_config"=w763) -> ("connection ID"=w781:refnum<k5>, "Connexion"=→"Connexion":bool, "Lecture"=→"Lecture":bool, "Écriture"=→"Écriture":bool, "Error OUT"=w779:errorcluster)  [unwired: 7 in]
              n548 = call <vilib>:"Close Config Data.vi"("error in (no error)"=w775, "refnum"=w774) -> ()  [unwired: 8 in, 2 out]
              n549 = local read "Hexapod VRN"() -> (w783:refnum<visa-resource-name>)
              n550 = case shown="Erreur" w779 {
                frame No Error {
                }
                frame Error {
                  n551 = One Button Dialog(message="Erreur lors de la connexion\nà l'hexapode-console.") -> ()  [unwired: 1 in, 1 out]
                }
              }
              n552 = Type Cast(type=w767, x=w781) -> (*(type *) &x=w780:string)
              n553 = Type Cast(type=w783, x=w780) -> (*(type *) &x=w782:refnum<visa-resource-name>)
              n554 = local write "Hexapod VRN"(w782) -> ()
            }
          }
          "PrAMS + Hexapode" <- w737
        }
      }
    }
    frame #6 {
      # "Étape 6 de l'initialisation"
      # "Configure les paramètres par défaut de PrAMS et Hexapode-Console"
      n555 = case shown="Vrai" w790 {
        frame False {
        }
        frame True {
          n556 = flat-sequence {
            frame #0 {
              w791 = u16 1 items=["Initialisation", "Retirer la lame séparatrice du faisceau", "Mettre la lame séparatrice dans le faisceau"] ("SpliterSelector")
              n557 = local write "SpliterSelector"(w791) -> ()
            }
            frame #1 {
              n558 = local read "path_config"() -> (w794:path)
              n559 = local read "PrAMS VRN"() -> (w803:refnum<visa-resource-name>)
              n560 = local read "Binning"() -> (w798:u16)
              n561 = local read "PrAMS Error"() -> (w801:errorcluster)
              n562 = local read "Signature"() -> (w802:u32)
              n563 = local read "ROIWidth"() -> (w797:u16)
              n564 = local read "ROIHeight"() -> (w796:u16)
              n565 = local read "ROIXOffset"() -> (w799:u16)
              n566 = local read "ROIYOffset"() -> (w800:u16)
              n567 = Build Path(base path=w794, name or relative path=path "command.ini" ("command.ini")) -> (appended path=w792:path)
              n568 = call "SAOMM-FalconFixer_patched.vi"("PRAMMS VRN"=w803, "ROIYOffset"=w800, "ROIXOffset"=w799, "Binning"=w798, "command.ini"=w792, "Signature"=w802, "PRAMMS Error"=w801, "ROIWidth"=w797, "ROIHeight"=w796) -> ("Error"=w795:bool)  [unwired: 6 in]
              n569 = case shown="Vrai" w795 {
                frame False {
                }
                frame True {
                  n570 = One Button Dialog(message="Une erreur est survenue lors de la configuration\nde la caméra de guidage.  Il se peut que certaines\nfonctionnalités ne soient pas disponibles.") -> ()  [unwired: 1 in, 1 out]
                }
              }
            }
            frame #2 {
              w805 = "emtAcknowlegment"
              n571 = local read "MessageType"() -> (w806:cluster{string[], u32[]})
              n572 = local read "Hexapod VRN"() -> (w820:refnum<visa-resource-name>)
              n573 = local read "PrAMS Error"() -> (w817:errorcluster)
              n574 = Type Cast(type=refnum<k5> refnum ("connection ID"), x=w820) -> (*(type *) &x=w822:refnum<k5>)
              n575 = local read "Signature"() -> (w813:u32)
              n576 = call-poly "SAOMM-Num2littleEndian.vi"("Number"="DefaultUAxisOffset") -> ("LiitleEndianedData"=w812:u8[])  [unwired: 14 in]
              n577 = call-poly "SAOMM-Num2littleEndian.vi"("Number"="DefaultVAxisOffset") -> ("LiitleEndianedData"=w811:u8[])  [unwired: 14 in]
              n578 = call "SendSET-NoListener.vi"("connection ID"=w822, "CommandArray"=w806, "ExpectedAnswer"=w805, "Signature"=w813, "Error IN"=w817, "Active SET"="emtSetUAxisOffset", "Value (little endianed byte array)"=w812) -> ("connection ID (dup)"=w815:refnum<k5>, "Succes"=→"SetUOffset":bool, "Error OUT"=w816:errorcluster)  [unwired: 6 in]
              n579 = call "SendSET-NoListener.vi"("connection ID"=w815, "CommandArray"=w806, "ExpectedAnswer"=w805, "Signature"=w813, "Error IN"=w816, "Active SET"="emtSetVAxisOffset", "Value (little endianed byte array)"=w811) -> ("Succes"=→"SetVOffset":bool, "Error OUT"=w814:errorcluster)  [unwired: 6 in, 1 out]
              n580 = local write "PrAMS Error"(w814) -> ()
            }
          }
        }
      }
    }
    frame #7 {
      # "- Ajustement des paramètres instrumentauux\n- Calcul des astrométries initiales\n- Initialisation des périphériques"
      n581 = case shown="Vrai" w823 {
        frame False {
        }
        frame True {
          n582 = flat-sequence {
            tunnel: [TRUE] -> w827
            tunnel: w827 -> [w869]
            tunnel: [TRUE] -> w826
            tunnel: w826 -> [w911]
            tunnel: [TRUE] -> w825
            tunnel: w825 -> [w943]
            tunnel: [TRUE] -> w824
            frame #0 {
              # "Argh :("
              # "Fais la première commande #25 pour obtenir les infos du TCS, envoie la commande \"STOP\",\npuis force le TCS en mode \"EST\""
              n583 = control-ref of="TCS actif"() -> (w836:refnum<vi>)
              n584 = call "Fractional-Year.vi"() -> ("Fractional Year"=w833:dbl)  [unwired: 15 in]
              n585 = local read "TCS VRN"() -> (w837:refnum<visa-resource-name>)
              n586 = local read "dflt-EQX"() -> (w832:dbl)
              n587 = Build Array(w833) -> (w834:dbl[])
              n588 = call "EXCOM-CMD.vi"("VRN IN"=w837, "Bool Refnum"=w836, "Commande #"=22, "Args"=w834) -> ("VRN OUT"=w838:refnum<visa-resource-name>)  [unwired: 9 in, 2 out]
              n589 = call "EXCOM-25-EQ.vi"("VISA resource name"=w838, "Bool Refnum"=w836, "Display Equinox"=w832) -> ("HA"=w845:dbl, "RA"=w846:dbl, "Rotateur"=w830:dbl, "DEC"=w847:dbl, "Dome"=w853:dbl, "Epoque"=w848:dbl, "Focus"=w852:dbl, "VISA resource name dup"=w855:refnum<visa-resource-name>, "Masse d'air"=w849:dbl, "Temps Sidéral"=w850:dbl, "Temps Universel"=w851:dbl, "Année"=w854:dbl, "Error OUT"=w856:errorcluster)  [unwired: 2 in, 2 out]
              n590 = local write "RA Tel"(w846) -> ()
              n591 = local write "DEC Tel"(w847) -> ()
              n592 = local write "RotationTCS"(w830) -> ()
              n593 = local write "Angle Hor."(w845) -> ()
              n594 = local write "Dectmp"(w847) -> ()
              n595 = local write "Epoch Tel"(w848) -> ()
              n596 = local write "Coupole"(w853) -> ()
              n597 = local write "RAtmp"(w846) -> ()
              n598 = local write "Air Mass"(w849) -> ()
              n599 = local write "AnnéeRL"(w854) -> ()
              n600 = local write "LST"(w850) -> ()
              n601 = local write "UTC"(w851) -> ()
              n602 = local write "Foyer"(w852) -> ()
              n603 = call "SerialCommError.vi"("VISA IN"=w855, "error IN"=w856) -> ("VISA OUT"=w857:refnum<visa-resource-name>, "Error"=w840:bool, "error OUT"=w844:errorcluster)  [unwired: 11 in]
              n604 = Negate(x=w830) -> (-x=w829:dbl)
              n605 = expression code="x+90"(w829) -> (w828:dbl)
              n606 = case shown="Vrai" w840 {
                tunnel: w850 -> [_ w861]
                tunnel: w848 -> [_ w860]
                tunnel: w847 -> [_ w859]
                tunnel: w846 -> [_ w858]
                frame False {
                }
                frame True {
                  n607 = call "Object_properties.vi"("Target RA"=w858, "Target DEC"=w859, "Target Epoch"=w860, "Sideral Time"=w861) -> ("NO RA"=w862:string, "NO DEC"=w863:string, "NO Epoch"=w865:dbl, "NO HA"=w864:dbl, "NO AM"=w866:dbl)  [unwired: 7 in]
                  n608 = local write "NO epoch"(w865) -> ()
                  n609 = local write "NO AM"(w866) -> ()
                  n610 = local write "NO HA"(w864) -> ()
                  n611 = local write "N.O. Déc."(w863) -> ()
                  n612 = local write "N.O. A.D."(w862) -> ()
                }
              }
              n613 = control-ref of="TCS actif"() -> (w839:refnum<vi>)
              n614 = local write "RotationEffective"(w828) -> ()
              n615 = call "EXCOM-CMD.vi"("VRN IN"=w857, "Bool Refnum"=w839, "Commande #"=13, "Error IN"=w844) -> ("VRN OUT"=w842:refnum<visa-resource-name>, "Error OUT"=w841:errorcluster)  [unwired: 9 in, 1 out]
              n616 = local write "TCS VRN"(w842) -> ()
              n617 = local write "TCS Error"(w841) -> ()
            }
            frame #1 {
              # "Demande l'instruments et synchronise Starry Night ..."
              # "Synchronise les coordonnées de StarryNight avec celle du télescope"
              n618 = local read "Instrument Actuel"() -> (w903:string)
              n619 = local read "SkipChoixInstr"() -> (w867:bool)
              n620 = local read "instruments.ini"() -> (w894:path)
              n621 = call "InstrChoice.vi"("Instrument IN"=w903, "SkipChoixInstr"=w867, "instruments.ini"=w894, "DisallowUndo"=TRUE) -> ("This VI's Path"=w888:path, "Instrument OUT"=w902:string, "FoV"=→"FOV":dbl, "foynom"=→"Foyer à 0°":i32, "atherm"=→"Ath_coef":dbl, "exclusion"=→"path_exclusion":path, "collim"=w871:path)  [unwired: 8 in, 1 out]
              "Instrument Actuel" <- w902
              n622 = Open VI Reference(vi path=w888) -> (vi reference=w878:refnum<vi>, error out=w877:errorcluster)  [unwired: 5 in]
              n623 = property class="VI"(reference=w878, error in=w877) -> (reference out=w882:refnum<vi>, error out=w881:errorcluster, "Front Panel.Open"=w880:bool)
              n624 = local read "Calib VRN"() -> (w892:refnum<visa-resource-name>)
              n625 = local read "Epoch Tel"() -> (w897:dbl)
              n626 = local read "RA Tel"() -> (w895:dbl)
              n627 = local read "DEC Tel"() -> (w896:dbl)
              n628 = Automation Open(Automation Refnum=refnum<k7> refnum ("ScopeSim._Telescope")) -> (Automation Refnum=w884:refnum<k7>)  [unwired: 3 in, 1 out]
              n629 = case shown="Faux" w880 {
                tunnel: w882 -> [_ w908]
                tunnel: w881 -> [w905 w907]
                tunnel: [w905 w906] -> w879
                frame False {
                }
                frame True {
                  n630 = invoke class="VI" method="FA.Fermer"(reference=w908, error in=w907) -> (error out=w906:errorcluster)  [unwired: 1 in, 2 out]
                }
              }
              n631 = local write "ActiveLUT"(w871) -> ()
              n632 = call "Controle_des_lampe.vi"("VISA resource name"=w892, "Status In"=bool[] [FALSE, FALSE, FALSE]) -> ("Status Out"=→"Status lamp":bool[])  [unwired: 2 out]
              n633 = Current VI's Menubar() -> (w901:refnum<k9>)
              n634 = call "Set_SN_Coords.vi"("Coords EPOCH"=w897, "input_DEC"=w896, "input_RA"=w895, "ScopeSim._Telescope"=w884) -> ("precessed_DEC"=w886:dbl, "precessed_RA"=w887:dbl)  [unwired: 6 in]
              n635 = global write "Globals.vi" "ScopeSim._Telescope"(w884) -> ()
              n636 = local write "VI Reference Error"(w879) -> ()
              n637 = Set Menu Item Info(6:TRUE ("coché"), 7:w902, 11:w901) -> (0:w889:errorcluster)  [unwired: 4 in, 1 out]
              n638 = local write "Dectmp"(w886) -> ()
              n639 = local write "RAtmp"(w887) -> ()
              n640 = call "SAOMM-XML2LUT.vi"("Path"=w871) -> ("NominalPositions"=w870:dbl[])  [unwired: 13 in, 1 out]
              n641 = local write "Menu Error"(w889) -> ()
              n642 = Index Array(array=w870) -> (element #3=w876:dbl, element #4=w875:dbl, element #5=w874:dbl, element #6=w873:dbl, element #7=w872:dbl)  [unwired: 7 in, 2 out]
              n643 = local write "Nominal Y"(w875) -> ()
              n644 = local write "Nominal X"(w876) -> ()
              n645 = local write "Nominal Z"(w874) -> ()
              n646 = local write "Nominal V"(w872) -> ()
              n647 = local write "Nominal U"(w873) -> ()
              "Initialisation TCS" <- w869
            }
            frame #2 {
              # "Initialisation des tables de guidages et de la connexion au simulateur de TELESCOPE\n\n possiblement qu'il faudra ajouter l'origine automatique des systèmes SAOMM"
              n648 = local read "Table VRN"() -> (w914:refnum<visa-resource-name>)
              n649 = local read "vitesse lente"() -> (w918:dbl)
              n650 = local read "accelleration"() -> (w916:dbl)
              n651 = control-ref of="Table actif"() -> (w915:refnum<vi>)
              n652 = local read "vitesse rapide"() -> (w917:dbl)
              n653 = local read "ActiveStages"() -> (w909:string[])
              "ActiveStages" <- w909
              n654 = for {
                tunnel: w909 -> [w925] mode=indexing
                tunnel: w918 -> [w926]
                tunnel: w917 -> [w927]
                tunnel: w916 -> [w928]
                tunnel: w915 -> [w929]
                tunnel: w914 -> [w932]
                tunnel: [w931] -> w913
                tunnel: [w930] -> w912
                n655 = call "Newmark-SetSpeed.vi"("Table VRN"=w932, "StageTAG"=w925, "Bool Refnum"=w929, "Vitesse Lente"=w926, "Vitesse Rapide"=w927, "Accélération"=w928) -> ("Table VRN OUT"=w931:refnum<visa-resource-name>, "Error OUT"=w930:errorcluster)  [unwired: 7 in, 1 out]
              }
              n656 = call "Newmark-QueryPosition.vi"("Table VRN IN"=w913, "Bool Refnum"=w915, "Error IN"=w912) -> ("X Axis"=w921:dbl, "Y Axis"=w920:dbl, "Table VRN OUT"=w923:refnum<visa-resource-name>, "Z Axis"=w919:dbl, "Error OUT"=w922:errorcluster)  [unwired: 5 in, 3 out]
              n657 = property on="Origine" class="Bool (strict)"("Blinking"=TRUE) -> ()  [unwired: 2 in, 2 out]
              n658 = local write "Position Z"(w919) -> ()
              n659 = local write "Position X"(w921) -> ()
              n660 = local write "Position Y"(w920) -> ()
              n661 = local write "Table VRN"(w923) -> ()
              n662 = local write "Table Error"(w922) -> ()
              "Choix de l'insturment" <- w911
            }
            frame #3 {
              w936 = 0.0
              w957 = u16 0 items=["Square", "Circle"] ("Ring")
              # "Invert X"
              # "Époque DSS et USNO"
              # "Seul le champ est approximé, dans un avenir lointain\non pourra tenir compte de la distorsion en ajoutant\nla structure de distortion décrite dans Calabretta et al 2004"
              n663 = local read "MirFOV"() -> (w935:dbl)
              n664 = local read "LimXPesto"() -> (w934:dbl)
              n665 = local read "Miroir"() -> (w938:dbl)
              n666 = local read "BrasPesto"() -> (w933:bool)
              n667 = local read "arcsec/pulse"() -> (w960:dbl)
              n668 = local read "CentreTel X"() -> (w966:dbl)
              n669 = local read "CentreTel Y"() -> (w967:dbl)
              n670 = local read "Reference X"() -> (w965:dbl)
              n671 = local read "Reference Y"() -> (w964:dbl)
              n672 = local read "RA Tel"() -> (w962:dbl)
              n673 = local read "DEC Tel"() -> (w961:dbl)
              n674 = local read "MirVig"() -> (w939:dbl)
              n675 = local read "RotationEffective"() -> (w941:dbl)
              n676 = local read "Représentation"() -> (w946:dbl)
              n677 = local read "Epoch Tel"() -> (w952:dbl)
              n678 = local read "FOV"() -> (w956:dbl)
              n679 = Bundle("MirVig"=w939, w936, w936, "Miroir"=w938, "MirFOV"=w935, "LimXPesto"=w934, "BrasPesto"=w933) -> (w937:T25)  [unwired: 1 in]
              n680 = call "Set_field_astrometry.vi"("Cen x (pas)"=w966, "effective rotation (°)"=w941, "scale (\"/pas)"=w960, "NaxisMax"=500000, "Cen y (pas)"=w967, "Use Center?"=FALSE, "Ref x (pas)"=w965, "Ref y (pas)"=w964, "RA (HH:MM:SS.S)"=w962, "DEC(DD:MM:SS)"=w961, "Inversion Cluster"=T20 {"Invert Angle"=FALSE, "Invert X"=TRUE, "Invert Y"=FALSE}) -> ("Field Astrometry"=w953:T4, "Table Astrometry"=w954:T4)  [unwired: 3 in]
              "FieldAstrom" <- w953
              n681 = call "draw_field.vi"("Field_Astrometry"=w953, "FOV"=w956, "Ring"=w957, "Table_Astrometry"=w954, "Ues Constant Size ?"=TRUE, "margin/size"=w946, "MirrorAvatar"=w937) -> ("TableXYPos"=w947:cluster{dbl[], dbl[]}[], "X Scale.Range"=w958:T26, "ImgDEC"=w940:dbl, "ImgRA"=w950:dbl, "Y Scale.Range"=w959:T26)  [unwired: 4 in]
              n682 = local write "TableAstrom"(w954) -> ()
              n683 = call "precess.vi"("Eq2"=2000.0, "Eq1"=w952, "DEC 1"=w940, "RA 1"=w950) -> ("DEC 2"=w948:dbl, "RA 2"=w949:dbl)
              n684 = local write "DEC-Champ"(w948) -> ()
              n685 = property on="TableXYPos" class="GraphXY (strict)"("Value"=w947, "XScale.Range"=w958, "YScale.Range"=w959) -> ()  [unwired: 2 in, 2 out]
              n686 = local write "RA-Champ"(w949) -> ()
              "Vitesse des tables" <- w943
            }
          }
          "Astrométries" <- w824
        }
      }
    }
    frame #8 {
      # "Boucle principale du programme"
      n687 = case shown="Vrai" w969 {
        frame False {
        }
        frame True {
          (unwired) TRUE
          # "Hexapode Listener"
          n688 = control-ref of="PrAMS actif"() -> (w984:refnum<vi>)
          n689 = Tick Count (ms)() -> (millisecond timer value=w985:u32)
          n690 = Tick Count (ms)() -> (millisecond timer value=w986:u32)
          n691 = control-ref of="HexaCons actif"() -> (w983:refnum<vi>)
          n692 = while {
            stop <- w987 stop-if-true
            n693 = local read "Cx"() -> (w989:bool)
            n694 = case shown="Faux" w989 {
              selector: w989 -> [_ w1015]
              tunnel: [w1005 w1015] -> w988
              frame False {
                # "Si on n'est pas connecté, on fait une tentative ..."
                n695 = flat-sequence {
                  tunnel: [w1006] -> w1004
                  tunnel: [w1008] -> w1005
                  tunnel: w1004 -> [_]
                  frame #0 {
                    n696 = local read "cRIO_commID"() -> (w1007:refnum<k5>)
                    n697 = TCP Close Connection(connection ID=w1007) -> (error out=w1006:errorcluster)  [unwired: 2 in, 1 out]
                  }
                  frame #1 {
                    n698 = local read "cRIO address"() -> (w1010:string)
                    n699 = TCP Open Connection(address=w1010, remote port or service name=u16 8088, timeout ms (60000)=5000) -> (connection ID=w1009:refnum<k5>, error out=w1013:errorcluster)  [unwired: 2 in]
                    n700 = local write "cRIO_commID"(w1009) -> ()
                    n701 = Unbundle By Name(w1013) -> ("status"=w1012:bool)
                    n702 = Not(x=w1012) -> (.not. x?=w1008:bool)
                    n703 = local write "Cx"(w1008) -> ()
                  }
                }
              }
              frame True {
              }
            }
            n704 = case shown="Vrai" w988 {
              frame False {
                w990 = 0.0 ("indic-T-out")
                n705 = local write "indic-Tm"(w990) -> ()
                n706 = local write "indic-T-struct"(w990) -> ()
                n707 = local write "indic-T-out"(w990) -> ()
                n708 = local write "indic-T-in"(w990) -> ()
                n709 = local write "indic-H-out"(w990) -> ()
                n710 = local write "indic-H-in"(w990) -> ()
              }
              frame True {
                n711 = local read "cRIO_commID"() -> (w1002:refnum<k5>)
                n712 = call "TCP-read.vi"("timeout (5000)"=60000, "connection ID"=w1002) -> ("error out"=w994:errorcluster, "data out"=w1003:string)  [unwired: 1 in, 1 out]
                n713 = Unbundle By Name(w994) -> ("status"=w993:bool)
                n714 = call "line2array.vi"("data-line"=w1003) -> ("data-array"=w1001:dbl[])  [unwired: 2 out]
                n715 = Not(x=w993) -> (.not. x?=w992:bool)
                n716 = local write "Cx"(w992) -> ()
                n717 = Index Array(array=w1001) -> (element #1=→"indic-T-out":dbl, element #2=→"indic-H-out":dbl, element #3=→"indic-T-in":dbl, element #4=→"indic-H-in":dbl, element #7=→"indic-Tm":dbl, element #8=→"indic-T-struct":dbl)  [unwired: 9 in, 3 out]
              }
            }
            n718 = local read "Quit"() -> (w987:bool)
          }
          n719 = while {
            tunnel: [w1178] -> w977
            stop <- w1178 stop-if-true
            # "ErrorDEC en Secondes d'arc ...."
            # "ErrorRA en Secondes d'arc ...."
            # "Applique la correction si le délai est respecté et\nque la valeur de l'erreur totale est plus grande que\nle treshold."
            # "Évalue s'il faut envoyer une commande au relais de guidage.\nEn fonction du mode choisi ..."
            n720 = local read "Mode"() -> (w1187:u16)
            n721 = case shown="4" w1187 {
              tunnel: [w1190 w1194 w1213 w1233] -> w1184
              tunnel: [w1190 w1193 w1215 w1232] -> w1185
              tunnel: [FALSE w1206 w1225 w1231] -> w1177
              tunnel: [FALSE FALSE FALSE w1231] -> w1170
              frame Default {
                w1190 = 0.0 ("mean")
              }
              frame 0, 1 {
                # "Oh, c'est pas propre ici ... le (-1) a été mis parce\nque comme un gros épais ... j'ai inversé RA/DEC et\nNS/EW dans l'autre boucle ..."
                # "Ne marchera pour une étoile qui serait près de RA=00h00m00s ou RA=23h59m59s"
                # "Opération Fixe ou Asservissement Passif"
                n722 = local read "GuiderAstrom"() -> (w1203:T4)
                n723 = local read "LastProcID"() -> (w1207:u64)
                n724 = local read "CorrID"() -> (w1208:u64)
                n725 = local read "XCentroid"() -> (w1205:dbl)
                n726 = local read "YCentroid"() -> (w1204:dbl)
